vi "Chroma 1905x Series Configure Hipot Low Limit Query.vi"(4 "Mode":T2 items=["AC", "DC"], 8 "error in (no error)":errorcluster, 9 "Step":T1=1 min=1 max=99 step=1, 11 "VISA resource name":refnum<visa-resource-name>) -> (0 "error out":errorcluster, 3 "VISA resource name out":refnum<visa-resource-name>)   [LabVIEW 2025]
uses:
  Type Def/modes AC DC--control.ctl
  step--control.ctl
panel:
  out "Low value [A]":string
  # "Configure Hipot Low Limit"
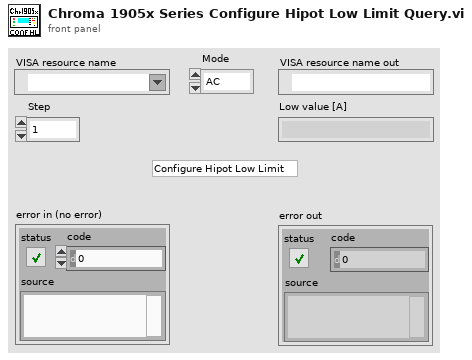
[diagram p1: front panel]
types:
  T1 = typedef "step--control.ctl" = u8
  T2 = typedef "modes AC DC--control.ctl" = i32
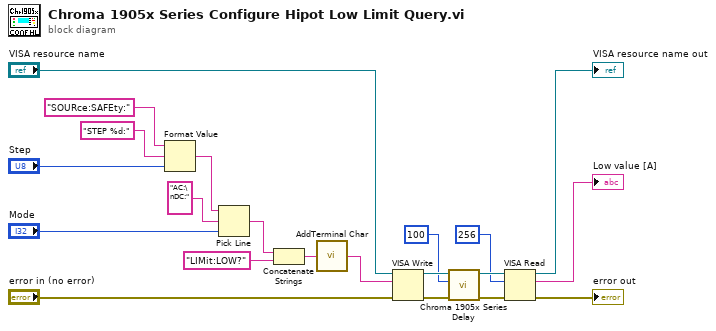
[diagram p0: block diagram]
diagram:
  n1 = Format Value(string ("")="SOURce:SAFEty:", format string="STEP %d:", value (0)="Step") -> (output string=w16:string)
  n2 = Pick Line(string ("")=w16, multi-line string="AC:\nDC:", line index="Mode") -> (output string=w2:string)
  n3 = Concatenate Strings(w2, "LIMit:LOW?" ("format string")) -> (w1:string)
  n4 = call "AddTerminal Char.vi"("Cmd string"=w1) -> ("Concatenated String"=w8:string)  [unwired: 4 in]
  n5 = VISA Write(VISA resource name="VISA resource name", write buffer=w8, error in (no error)="error in (no error)") -> (VISA resource name out=w13:refnum<visa-resource-name>, error out=w15:errorcluster)  [unwired: 1 out]
  n6 = call "Chroma 1905x Series Delay.vi"("error in (no error)"=w15, "Time Delay [ms]"=u32 100 ("Time Delay ms"), "VISA resource name"=w13) -> ("error out"=w14:errorcluster, "VISA resource name 2"=w12:refnum<visa-resource-name>)  [unwired: 7 in]
  n7 = VISA Read(VISA resource name=w12, byte count=u32 256, error in (no error)=w14) -> (VISA resource name out=→"VISA resource name out":refnum<visa-resource-name>, read buffer=→"Low value [A]":string, error out=→"error out":errorcluster)  [unwired: 1 out]
